vi "imaging_or_resting.vi"(11 "Scan counters":T1 {"Current part of waveform" items=["Imaging", "Settling", "Resting"]}) -> (1 "Currently at resting part?":bool, 2 "Currently at settling part?":bool, 3 "Currently at imaging part?":bool)   [LabVIEW 2011]
uses:
  typedefs/scan_counters_cluster.ctl
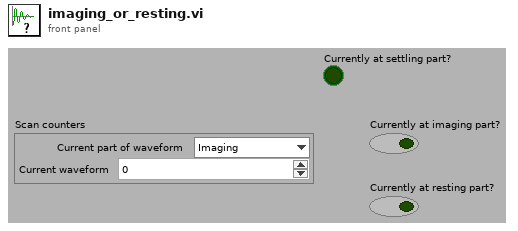
[diagram p1: front panel]
types:
  T1 = typedef "scan_counters_cluster.ctl" = cluster{"Current part of waveform":u8, "Current waveform":u16}
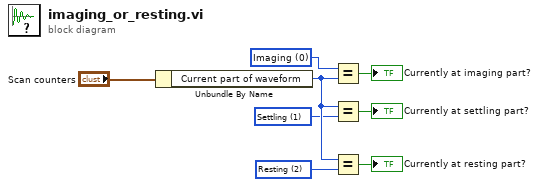
[diagram p0: block diagram]
diagram:
  w2 = u8 1 items=["Imaging", "Settling", "Resting"] ("Current part of waveform")
  w8 = u8 0 items=["Imaging", "Settling", "Resting"] ("Current part of waveform")
  w7 = u8 2 items=["Imaging", "Settling", "Resting"] ("Current part of waveform")
  n1 = Unbundle By Name("Scan counters") -> ("Current part of waveform"=w3:u8)
  n2 = Equal?(x=w8, y=w3) -> (x = y?=→"Currently at imaging part?":bool)
  n3 = Equal?(x=w3, y=w2) -> (x = y?=→"Currently at settling part?":bool)
  n4 = Equal?(x=w3, y=w7) -> (x = y?=→"Currently at resting part?":bool)
